vi "rs3 start tare.vi"(7 "error in (no error)":errorcluster, 9 "Tare depth":dbl, 10 "device in":u64) -> (0 "error out":errorcluster, 1 "error":u64, 3 "Device out":u64, 4 "result (0=success)":i32)   [LabVIEW 2017, in "libRealSense3.lvlib"]
doc: "Start the on-chip tare calibration, where user inputs known ground-truth absolute distance to a wall. \nThis method calculated the average distance as the average of the full FOV. \nThe status of the results can be querried with Get Tare status, and the calibration can also be stored in flash using the Burn Tare Cal command."
uses:
  libRealSense3.lvlib
  realsense2.dll
panel:
  # "RS3 Start Tare Cal."
  # "(C) Intel Corp. 2019,  AGJ"
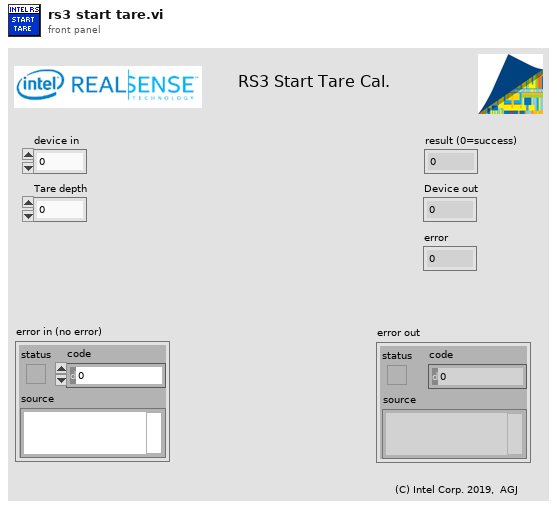
[diagram p1: front panel]
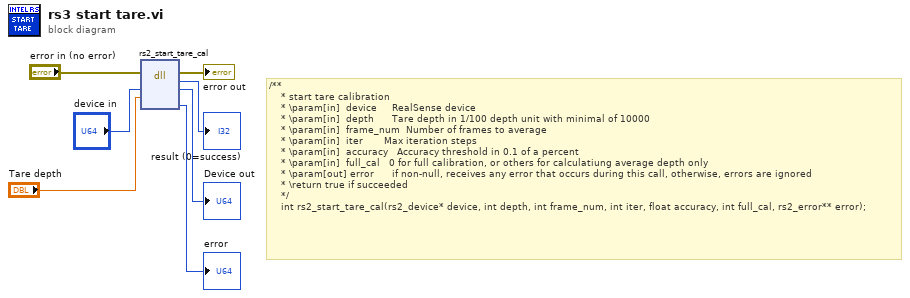
[diagram p0: block diagram]
diagram:
  # "/**\n    * start tare calibration\n    * \\param[in]  device     RealSense device\n    * \\param[in]  depth      Tare depth in 1/100 depth unit with minimal of 10000\n    * \\param[in]  frame_num  Number of frames to average   \n    * \\param[in]  iter       Max iteration steps\n    * \\param[in]  accuracy   Accuracy threshold in 0.1 of a percent\n    * \\param[in]  full_cal   0 for full calibration, or others for calculatiung average depth only\n    * \\param[out] error      if non-null, receives any error that occurs during this call, otherwise, errors are ignored\n    * \\return true if succeeded\n    */\n    int rs2_start_tare_cal(rs2_device* device, int depth, int frame_num, int iter, float accuracy, int full_cal, rs2_error** error);"
  n1 = dll-call lib="C:/Users/agrunnet/Documents/libRealSense6/realsense2.dll" fn="rs2_start_tare_cal"(error in="error in (no error)", "device"="device in", "tare depth"="Tare depth") -> (error out=→"error out":errorcluster, "result"=→"result (0=success)":i32, "device"=→"Device out":u64, "error"=→"error":u64)  [unwired: 4 in, 1 out]
